vi "myRIO v1.0 Write I2C.vi"(4 "Keep Bus Busy":bool, 6 "Slave Address (7-bit)":u8, 7 "Timeout ms (1000)":i32=1000, 8 "Error In (No Error)":errorcluster, 9 "Data to Write":u8[](array[numeric]), 10 "Channel":T1, 11 "myRIO Ref In":T2) -> (0 "error out":errorcluster, 3 "myRIO Ref Out":T2)   [LabVIEW 2021]
uses:
  <vilib>/myRIO/Common/Instrument Driver Framework/Utilities/typedefs/myRIO v1.0 Reference.ctl
  <vilib>/myRIO/Common/Instrument Driver Framework/Utilities/typedefs/Generic FPGA Reference.ctl
  <vilib>/myRIO/Common/Instrument Driver Framework/myRIO v1.0/I2C/typedefs/I2C Channels Enum.ctl
  <vilib>/myRIO/Common/Instrument Driver Framework/myRIO v1.0/I2C/typedefs/I2C Channels FPGA Reference.ctl
  <vilib>/rvi/errors/niLvFpgaAdjustHostInterfaceError.vi
  <vilib>/rvi/interface/nirviReadWriteControl/nirviReadWriteControl.xnode
  <vilib>/rvi/interface/Simulation/niFpgaSimulationCallBeginRW.vi
  NiFpgaLv.dll
panel:
  # "This VI writes an array of data to the SPI Data Out register (SPIn.SPDO) and reads an array of data from the SPI Data In register (SPIn.SPDI) for a particular SPI channel (n). The data is written/read one value at a time. Please see Block Diagram for details."
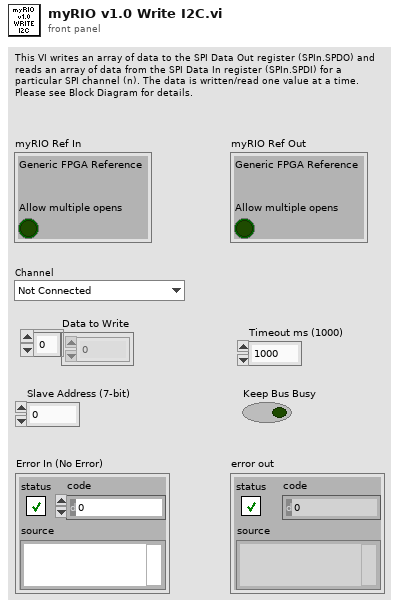
[diagram p1: front panel]
types:
  T1 = typedef "I2C Channels Enum.ctl" = enum16{"Not Connected", "A/I2C", "B/I2C", "I2C/I2C"}
  T2 = typedef "myRIO v1.0 Reference.ctl" = cluster{"Generic FPGA Reference":T3, "Allow multiple opens":bool}
  T3 = typedef "Generic FPGA Reference.ctl" = refnum<k20>
  T4 = typedef "I2C Channels FPGA Reference.ctl" = refnum<k20>
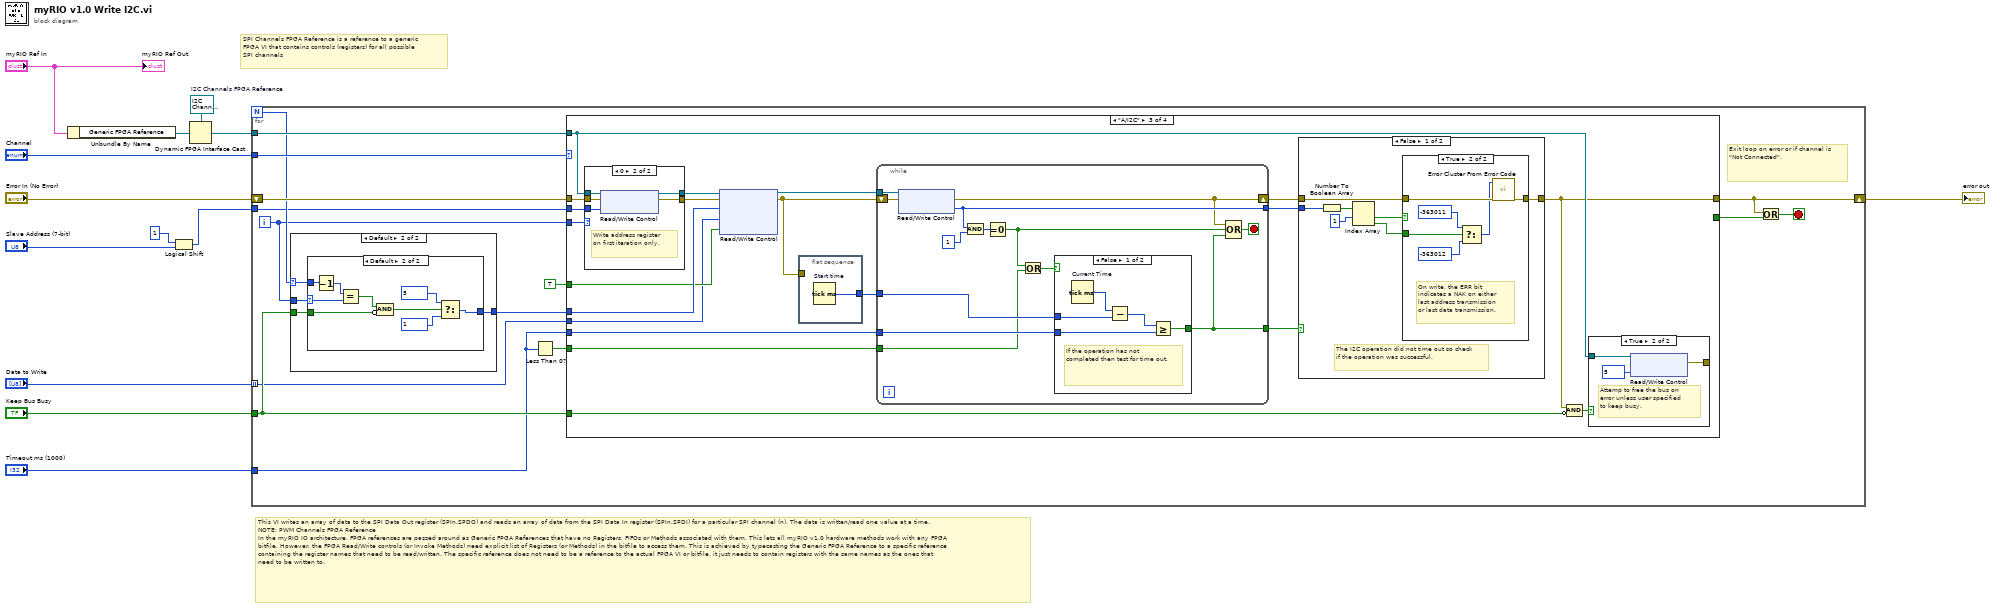
[diagram p0: block diagram]
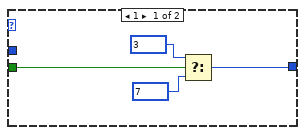
[diagram p2: hidden frame]
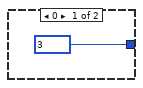
[diagram p3: hidden frame]
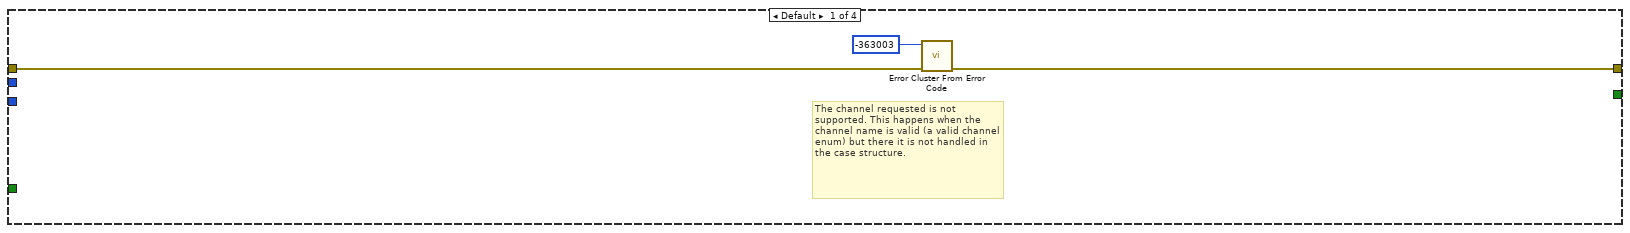
[diagram p4: hidden frame]
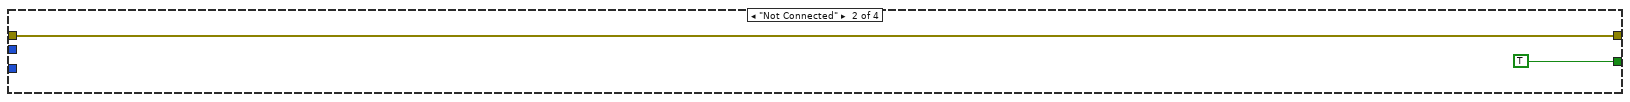
[diagram p5: hidden frame]
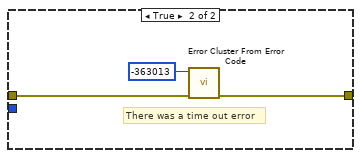
[diagram p7: hidden frame]
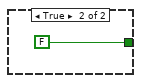
[diagram p10: hidden frame]
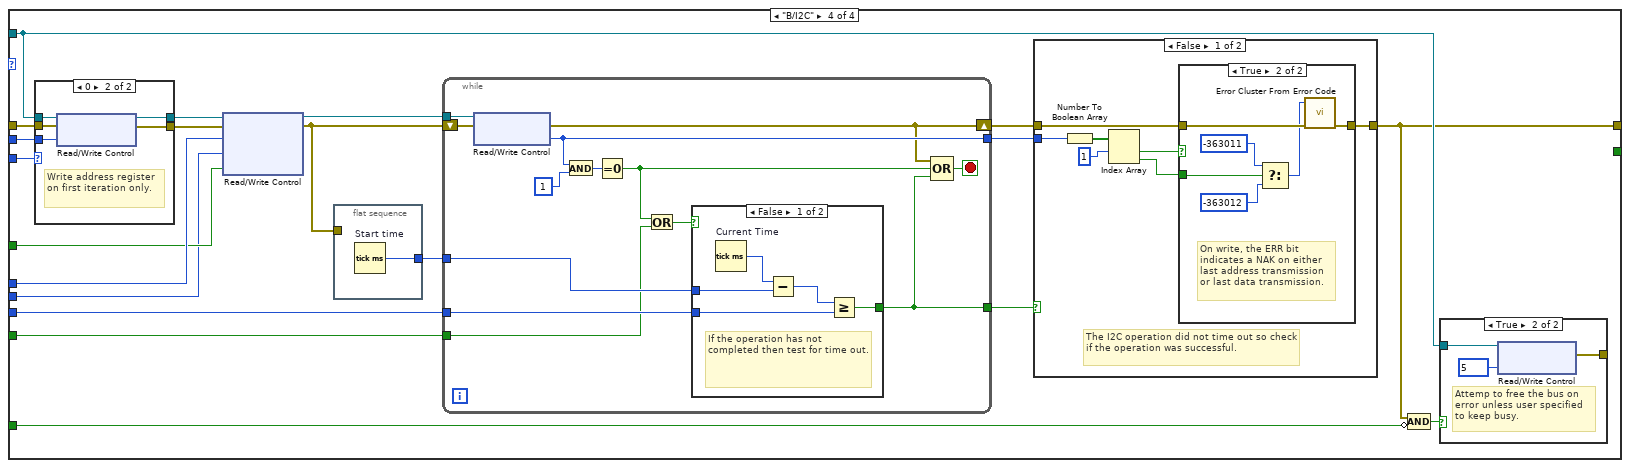
[diagram p11: hidden frame]
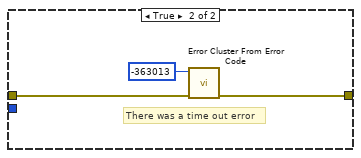
[diagram p13: hidden frame]
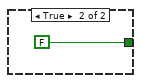
[diagram p16: hidden frame]
diagram:
  w11 = T4 refnum  # I2C Channels FPGA Reference
  # "This VI writes an array of data to the SPI Data Out register (SPIn.SPDO) and reads an array of data from the SPI Data In register (SPIn.SPDI) for a particular SPI channel (n). The data is written/read one value at a time.\nNOTE: PWM Channels FPGA Reference\nIn the myRIO IO architecture, FPGA references are passed around as Generic FPGA References that have no Registers, FIFOs or Methods associated with them. This lets all myRIO v1.0 hardware methods work with any FPGA bitfile. However, the FPGA Read/Write controls (or Invoke Methods) need explicit list of Registers (or Methods) in the bitfile to access them. This is achieved by typecasting the Generic FPGA Reference to a specific reference containing the register names that need to be read/written. The specific reference does not need to be a reference to the actual FPGA VI or bitfile, it just needs to contain registers with the same names as the ones that need to be written to."
  # "SPI Channels FPGA Reference is a reference to a generic FPGA VI that contains controls (registers) for all possible SPI channels"
  n1 = Unbundle By Name("myRIO Ref In") -> ("Generic FPGA Reference"=w2:T3)
  n2 = Logical Shift(y=i8 1, x="Slave Address (7-bit)") -> (x << y=w5:u8)
  n3 = Dynamic FPGA Interface Cast(Session In=w11, Type=w2) -> (Session Out=w6:T4)
  n4 = for {
    N -> [w23]
    tunnel: "Channel" -> [w27]
    shift-right: [w19] -> w8
    shift-left: "Error In (No Error)" -> [w28]
    tunnel: w6 -> [w26]
    tunnel: "Keep Bus Busy" -> [w20]
    tunnel: w5 -> [w22]
    tunnel: "Data to Write" -> [w16] mode=indexing
    tunnel: "Timeout ms (1000)" -> [w15]
    i -> [w21]
    stop <- w17 stop-if-true
    # "Exit loop on error or if channel is \"Not Connected\"."
    n5 = case shown="Default" w23 {
      selector: w23 -> [_ w34]
      tunnel: [w32 w35] -> w24
      tunnel: w21 -> [_ w36]
      tunnel: w20 -> [w30 w33]
      frame 1 {
        n6 = Select(t=u8 3 ("y"), s=w30, f=u8 7 ("y")) -> (s? t:f=w32:u8)
      }
      frame Default {
        n7 = case shown="Default" w36 {
          selector: w36 -> [_ w44]
          tunnel: [u8 3 ("y") w38] -> w35
          tunnel: w34 -> [_ w46]
          tunnel: w33 -> [_ w40]
          frame 0 {
          }
          frame Default {
            n8 = Decrement(x=w46) -> (x-1=w45:i32)
            n9 = Equal?(x=w45, y=w44) -> (x = y?=w41:bool)
            n10 = Compound Arithmetic op=AND(w41, invert w40) -> (w39:bool)
            n11 = Select(t=u8 5 ("y"), s=w39, f=u8 1 ("y")) -> (s? t:f=w38:u8)
          }
        }
      }
    }
    n12 = Less Than 0?(x=w15) -> (x < 0?=w14:bool)
    n13 = case shown="\"A/I2C\"" w27 {
      tunnel: w28 -> [w48 w51 w65 w132]
      tunnel: [w47 w51 w60 w127] -> w19
      tunnel: w26 -> [_ _ w62 w129]
      tunnel: w24 -> [_ _ w71 w138]
      tunnel: TRUE ("I2C0.GO") -> [_ _ w58 w125]
      tunnel: [_ TRUE _ _] -> w18
      tunnel: w22 -> [_ _ w64 w131]
      tunnel: w21 -> [_ _ w63 w130]
      tunnel: w20 -> [_ _ w61 w128]
      tunnel: w16 -> [_ _ w57 w124]
      tunnel: w15 -> [_ _ w54 w121]
      tunnel: w14 -> [_ _ w53 w120]
      frame Default {
        # "The channel requested is not supported. This happens when the channel name is valid (a valid channel enum) but there it is not handled in the case structure."
        n14 = call <vilib>:"Error Cluster From Error Code.vi"("error in (no error)"=w48, "error code (0)"=-363003) -> ("error out"=w47:errorcluster)  [unwired: 7 in]
      }
      frame "Not Connected" {
      }
      frame "A/I2C" {
        n15 = case shown="0" w63 {
          tunnel: [w94 w99] -> w67
          tunnel: [w93 w98] -> w66
          tunnel: w62 -> [w94 w97]
          tunnel: w65 -> [w93 w96]
          tunnel: w64 -> [_ w95]
          frame Default {
          }
          frame 0 {
            # "Write address register on first iteration only."
            n16 = xnode "Read/Write Control"("FPGA VI Reference In"=w97, "error in"=w96, "I2C.A.ADDR"=w95) -> ("FPGA VI Reference Out"=w99:T4, "error out"=w98:errorcluster)
          }
        }
        n17 = xnode "Read/Write Control"("FPGA VI Reference In"=w67, "error in"=w66, "I2C.A.CNTL"=w71, "I2C.A.DATO"=w57, "I2C.A.GO"=w58) -> ("FPGA VI Reference Out"=w70:T4, "error out"=w52:errorcluster)
        n18 = flat-sequence {
          tunnel: [w72] -> w56
          tunnel: w52 -> [_]
          frame #0 {
            n19 = Tick Count (ms) "Start time"() -> (millisecond timer value=w72:u32)
          }
        }
        n20 = while {
          tunnel: w70 -> [w111]
          shift-right: [w106] -> w69
          shift-left: w52 -> [w112]
          tunnel: [w107] -> w68
          tunnel: w56 -> [w105]
          tunnel: [w104] -> w55
          tunnel: w54 -> [w103]
          tunnel: w53 -> [w100]
          stop <- w108 stop-if-true
          n21 = xnode "Read/Write Control"("FPGA VI Reference In"=w111, "error in"=w112) -> ("error out"=w106:errorcluster, "I2C.A.STAT"=w107:u8)  [unwired: 1 out]
          n22 = And(x=w107, y=u8 1) -> (x .and. y?=w109:u8)
          n23 = Equal To 0?(x=w109) -> (x = 0?=w101:bool)
          n24 = Or(x=w101, y=w100) -> (x .or. y?=w102:bool)
          n25 = case shown="False" w102 {
            tunnel: w105 -> [w115 _]
            tunnel: [w114 FALSE] -> w104
            tunnel: w103 -> [w113 _]
            frame False {
              # "If the operation has not completed then test for time out."
              n26 = Tick Count (ms) "Current Time"() -> (millisecond timer value=w116:u32)
              n27 = Subtract(x=w116, y=w115) -> (x-y=w117:u32)
              n28 = Greater Or Equal?(x=w117, y=w113) -> (x >= y?=w114:bool)
            }
            frame True {
            }
          }
          n29 = Compound Arithmetic op=OR(w106, w101, w104) -> (w108:bool)
        }
        n30 = case shown="False" w55 {
          tunnel: w69 -> [w79 w88]
          tunnel: w68 -> [w78 _]
          tunnel: [w74 w87] -> w60
          frame False {
            # "The I2C operation did not time out so check if the operation was successful."
            n31 = Number To Boolean Array(number=w78) -> (Boolean array=w77:bool[])
            n32 = Index Array(array=w77, index #1=1 ("index")) -> (element #1=w76:bool, element #2=w73:bool)  [unwired: 1 in]
            n33 = case shown="True" w76 {
              tunnel: w79 -> [w80 w85]
              tunnel: [w80 w86] -> w74
              tunnel: w73 -> [_ w82]
              frame False {
              }
              frame True {
                # "On write, the ERR bit indicates a NAK on either last address transmission or last data transmission."
                n34 = Select(t=-363011, s=w82, f=-363012) -> (s? t:f=w83:i32)
                n35 = call <vilib>:"Error Cluster From Error Code.vi"("error in (no error)"=w85, "error code (0)"=w83) -> ("error out"=w86:errorcluster)  [unwired: 7 in]
              }
            }
          }
          frame True {
            # "There was a time out error"
            n36 = call <vilib>:"Error Cluster From Error Code.vi"("error in (no error)"=w88, "error code (0)"=-363013) -> ("error out"=w87:errorcluster)  [unwired: 7 in]
          }
        }
        n37 = Compound Arithmetic op=AND(w60, invert w61) -> (w59:bool)
        n38 = case shown="True" w59 {
          tunnel: w62 -> [_ w92]
          tunnel: [_ w90] -> _
          frame False {
          }
          frame True {
            # "Attemp to free the bus on error unless user specified to keep busy."
            n39 = xnode "Read/Write Control"("FPGA VI Reference In"=w92, "I2C.A.CNTL"=u8 5 ("I2C.C_0.CNTL")) -> ("error out"=w90:errorcluster)  [unwired: 1 in, 1 out]
          }
        }
      }
      frame "B/I2C" {
        n40 = case shown="0" w130 {
          tunnel: [w161 w166] -> w134
          tunnel: [w160 w165] -> w133
          tunnel: w129 -> [w161 w164]
          tunnel: w132 -> [w160 w163]
          tunnel: w131 -> [_ w162]
          frame Default {
          }
          frame 0 {
            # "Write address register on first iteration only."
            n41 = xnode "Read/Write Control"("FPGA VI Reference In"=w164, "error in"=w163, "I2C.B.ADDR"=w162) -> ("FPGA VI Reference Out"=w166:T4, "error out"=w165:errorcluster)
          }
        }
        n42 = xnode "Read/Write Control"("FPGA VI Reference In"=w134, "error in"=w133, "I2C.B.CNTL"=w138, "I2C.B.DATO"=w124, "I2C.B.GO"=w125) -> ("FPGA VI Reference Out"=w137:T4, "error out"=w119:errorcluster)
        n43 = flat-sequence {
          tunnel: [w139] -> w123
          tunnel: w119 -> [_]
          frame #0 {
            n44 = Tick Count (ms) "Start time"() -> (millisecond timer value=w139:u32)
          }
        }
        n45 = while {
          tunnel: w137 -> [w178]
          shift-right: [w173] -> w136
          shift-left: w119 -> [w179]
          tunnel: [w174] -> w135
          tunnel: w123 -> [w172]
          tunnel: [w171] -> w122
          tunnel: w121 -> [w170]
          tunnel: w120 -> [w167]
          stop <- w175 stop-if-true
          n46 = xnode "Read/Write Control"("FPGA VI Reference In"=w178, "error in"=w179) -> ("error out"=w173:errorcluster, "I2C.B.STAT"=w174:u8)  [unwired: 1 out]
          n47 = And(x=w174, y=u8 1) -> (x .and. y?=w176:u8)
          n48 = Equal To 0?(x=w176) -> (x = 0?=w168:bool)
          n49 = Or(x=w168, y=w167) -> (x .or. y?=w169:bool)
          n50 = case shown="False" w169 {
            tunnel: w172 -> [w182 _]
            tunnel: [w181 FALSE] -> w171
            tunnel: w170 -> [w180 _]
            frame False {
              # "If the operation has not completed then test for time out."
              n51 = Tick Count (ms) "Current Time"() -> (millisecond timer value=w183:u32)
              n52 = Subtract(x=w183, y=w182) -> (x-y=w184:u32)
              n53 = Greater Or Equal?(x=w184, y=w180) -> (x >= y?=w181:bool)
            }
            frame True {
            }
          }
          n54 = Compound Arithmetic op=OR(w173, w168, w171) -> (w175:bool)
        }
        n55 = case shown="False" w122 {
          tunnel: w136 -> [w146 w155]
          tunnel: w135 -> [w145 _]
          tunnel: [w141 w154] -> w127
          frame False {
            # "The I2C operation did not time out so check if the operation was successful."
            n56 = Number To Boolean Array(number=w145) -> (Boolean array=w144:bool[])
            n57 = Index Array(array=w144, index #1=1 ("index")) -> (element #1=w143:bool, element #2=w140:bool)  [unwired: 1 in]
            n58 = case shown="True" w143 {
              tunnel: w146 -> [w147 w152]
              tunnel: [w147 w153] -> w141
              tunnel: w140 -> [_ w149]
              frame False {
              }
              frame True {
                # "On write, the ERR bit indicates a NAK on either last address transmission or last data transmission."
                n59 = Select(t=-363011, s=w149, f=-363012) -> (s? t:f=w150:i32)
                n60 = call <vilib>:"Error Cluster From Error Code.vi"("error in (no error)"=w152, "error code (0)"=w150) -> ("error out"=w153:errorcluster)  [unwired: 7 in]
              }
            }
          }
          frame True {
            # "There was a time out error"
            n61 = call <vilib>:"Error Cluster From Error Code.vi"("error in (no error)"=w155, "error code (0)"=-363013) -> ("error out"=w154:errorcluster)  [unwired: 7 in]
          }
        }
        n62 = Compound Arithmetic op=AND(w127, invert w128) -> (w126:bool)
        n63 = case shown="True" w126 {
          tunnel: w129 -> [_ w159]
          tunnel: [_ w157] -> _
          frame False {
          }
          frame True {
            # "Attemp to free the bus on error unless user specified to keep busy."
            n64 = xnode "Read/Write Control"("FPGA VI Reference In"=w159, "I2C.B.CNTL"=u8 5 ("I2C.C_0.CNTL")) -> ("error out"=w157:errorcluster)  [unwired: 1 in, 1 out]
          }
        }
      }
    }
    n65 = Or(x=w19, y=w18) -> (x .or. y?=w17:bool)
  }
  "error out" <- w8
  "myRIO Ref Out" <- "myRIO Ref In"
